vi "Execute SQL (no return data).vi"(8 "error in (no error)":errorcluster, 9 "[disabled] return type (string)":string, 10 "sql (string)":string="SELECT * FROM employees;", 11 "database in":path=path "C:/labview/sqlite_dbManager/test/chinook.db") -> (0 "error out":errorcluster)   [LabVIEW 2020, in "sqlite3.lvlib"]
uses:
  sqlite3.lvlib
  sqlite/subvi/Error Converter (ErrCode or Status).vi
  sqlite/VIs/errstr.vi
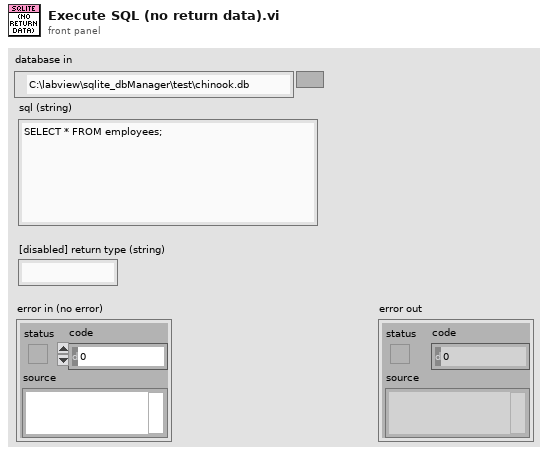
[diagram p1: front panel]
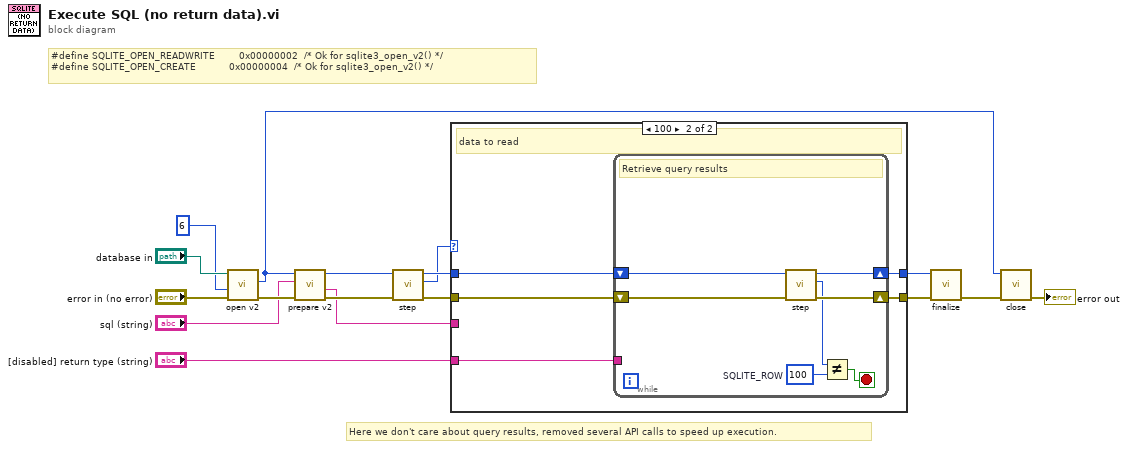
[diagram p0: block diagram]
diagram:
  # "#define SQLITE_OPEN_READWRITE        0x00000002  /* Ok for sqlite3_open_v2() */\n#define SQLITE_OPEN_CREATE           0x00000004  /* Ok for sqlite3_open_v2() */"
  # "Here we don't care about query results, removed several API calls to speed up execution."
  n1 = call "open v2.vi"("error in (no error)"="error in (no error)", "custom flags(rw/create)"=6 ("x .or. y?"), "filename"="database in") -> ("error out"=w15:errorcluster, "ppDb out"=w4:u64)  [unwired: 7 in]
  n2 = call "prepare v2.vi"("error in (no error)"=w15, "zSql"="sql (string)", "db"=w4) -> ("error out"=w13:errorcluster, "pzTail"=w1:string, "ppStmt out"=w6:u64)  [unwired: 6 in]
  n3 = call "step.vi"("error in (no error)"=w13, "para0"=w6) -> ("error out"=w11:errorcluster, "sqlite3_step"=w10:i32, "para0 out"=w12:u64)  [unwired: 7 in]
  n4 = case shown="100" w10 {
    tunnel: w12 -> [w19 w20]
    tunnel: w11 -> [w18 w21]
    tunnel: [w18 w23] -> w9
    tunnel: [w19 w24] -> w8
    tunnel: "[disabled] return type (string)" -> [_ w22]
    tunnel: w1 -> [_ _]
    frame 0, 101, Default {
      # "no data to read"
    }
    frame 100 {
      # "data to read"
      n5 = while {
        shift-right: [w31] -> w24
        shift-left: w20 -> [w25]
        shift-right: [w30] -> w23
        shift-left: w21 -> [w26]
        tunnel: w22 -> [_]
        stop <- w27 stop-if-true
        w28 = 100  # SQLITE_ROW
        # "Retrieve query results"
        n6 = call "step.vi"("error in (no error)"=w26, "para0"=w25) -> ("error out"=w30:errorcluster, "sqlite3_step"=w29:i32, "para0 out"=w31:u64)  [unwired: 7 in]
        n7 = Not Equal?(x=w29, y=w28) -> (x != y?=w27:bool)
      }
    }
  }
  n8 = call "finalize.vi"("error in (no error)"=w9, "pStmt"=w8) -> ("error out"=w3:errorcluster)  [unwired: 9 in]
  n9 = call "close.vi"("error in (no error)"=w3, "para0"=w4) -> ("error out"=→"error out":errorcluster)  [unwired: 9 in]
